vi "solar_excel Cell Range.vi"(10 "End (1,1 = 'A1')":cluster{"Row":u32, "Column":u32}, 11 "Start (1,1 = 'A1')":cluster{"Row":u32, "Column":u32}) -> (2 "End Cell":string, 3 "Start Cell":string, 5 "Same":bool)   [LabVIEW 2018]
doc: "This formats the Excel cell range as <letter><number> column & row pairs. (Ex: Col:2, Row:1 = 'B1')"
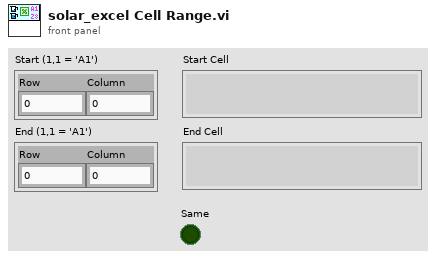
[diagram p1: front panel]
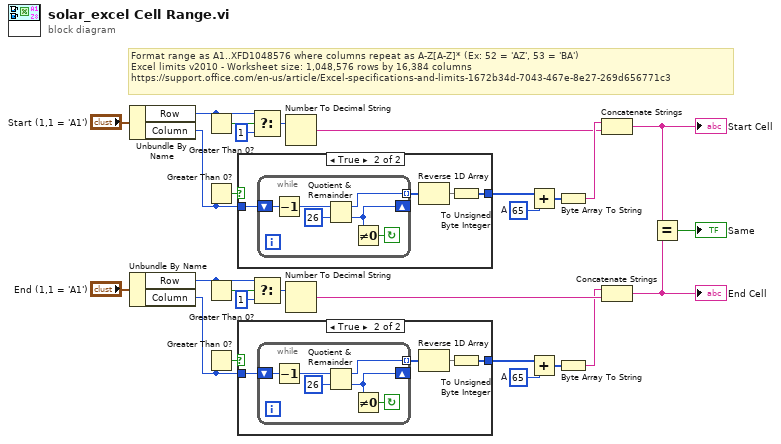
[diagram p0: block diagram]
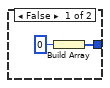
[diagram p2: hidden frame]
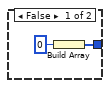
[diagram p3: hidden frame]
diagram:
  w7 = u8 65  # A
  w24 = u8 65  # A
  # "Format range as A1..XFD1048576 where columns repeat as A-Z[A-Z]* (Ex: 52 = 'AZ', 53 = 'BA')\nExcel limits v2010 - Worksheet size: 1,048,576 rows by 16,384 columns\nhttps://support.office.com/en-us/article/Excel-specifications-and-limits-1672b34d-7043-467e-8e27-269d656771c3"
  n1 = Unbundle By Name("Start (1,1 = 'A1')") -> ("Row"=w16:u32, "Column"=w21:u32)
  n2 = Unbundle By Name("End (1,1 = 'A1')") -> ("Row"=w15:u32, "Column"=w10:u32)
  n3 = Greater Than 0?(x=w16) -> (x > 0?=w19:bool)
  n4 = Greater Than 0?(x=w21) -> (x > 0?=w20:bool)
  n5 = Greater Than 0?(x=w15) -> (x > 0?=w12:bool)
  n6 = Greater Than 0?(x=w10) -> (x > 0?=w11:bool)
  n7 = case shown="True" w20 {
    tunnel: [w28 w31] -> w23
    tunnel: w21 -> [_ w30]
    frame False {
      n8 = Build Array(u8 0) -> (w28:u8[])
    }
    frame True {
      n9 = while {
        shift-right: [w36] -> _
        shift-left: w30 -> [w38]
        tunnel: [w35] -> w33 mode=indexing
        stop <- w37 continue-if-true
        n10 = Decrement(x=w38) -> (x-1=w34:u32)
        n11 = Quotient & Remainder(x=w34, y=u32 26) -> (x-y*floor(x/y)=w35:u32, floor(x/y)=w36:u32)
        n12 = Not Equal To 0?(x=w36) -> (x != 0?=w37:bool)
      }
      n13 = Reverse 1D Array(array=w33) -> (reversed array=w32:u32[])
      n14 = To Unsigned Byte Integer(number=w32) -> (unsigned 8bit integer=w31:u8[])
    }
  }
  n15 = case shown="True" w11 {
    tunnel: [w40 w43] -> w8
    tunnel: w10 -> [_ w42]
    frame False {
      n16 = Build Array(u8 0) -> (w40:u8[])
    }
    frame True {
      n17 = while {
        shift-right: [w48] -> _
        shift-left: w42 -> [w50]
        tunnel: [w47] -> w45 mode=indexing
        stop <- w49 continue-if-true
        n18 = Decrement(x=w50) -> (x-1=w46:u32)
        n19 = Quotient & Remainder(x=w46, y=u32 26) -> (x-y*floor(x/y)=w47:u32, floor(x/y)=w48:u32)
        n20 = Not Equal To 0?(x=w48) -> (x != 0?=w49:bool)
      }
      n21 = Reverse 1D Array(array=w45) -> (reversed array=w44:u32[])
      n22 = To Unsigned Byte Integer(number=w44) -> (unsigned 8bit integer=w43:u8[])
    }
  }
  n23 = Select(t=w16, s=w19, f=u32 1 ("t")) -> (s? t:f=w18:u32)
  n24 = Select(t=w15, s=w12, f=u32 1 ("t")) -> (s? t:f=w13:u32)
  n25 = Number To Decimal String(number=w18) -> (decimal integer string=w25:string)  [unwired: 1 in]
  n26 = Number To Decimal String(number=w13) -> (decimal integer string=w6:string)  [unwired: 1 in]
  n27 = Add(x=w23, y=w24) -> (x+y=w22:u8[])
  n28 = Add(x=w8, y=w7) -> (x+y=w9:u8[])
  n29 = Byte Array To String(unsigned byte array=w22) -> (string=w26:string)
  n30 = Byte Array To String(unsigned byte array=w9) -> (string=w5:string)
  n31 = Concatenate Strings(w26, w25) -> (w3:string)
  "Start Cell" <- w3
  n32 = Concatenate Strings(w5, w6) -> (w2:string)
  "End Cell" <- w2
  n33 = Equal?(x=w3, y=w2) -> (x = y?=→"Same":bool)
